vi "002 Panel Select.vi"(11 "Queue Ref In":T1={"UI"=refnum, "Message"=refnum, "Data"=refnum, "Caller"=refnum, "Name"="000 Common", "Data Path"=path "", "Class Path"=path "", "SubPanel"=refnum, "Project Name"="", "MNT"="", "Title"="", "Data Source"=refnum, "Queue List"={}, "VI"=refnum, "UE"=refnum}) -> ()   [LabVIEW 2020]
doc: "000001"
uses:
  Alin/QMH/000 Module Data Type.ctl
  Alin/QMH/Queue Message.ctl
  0007 Controls/Panel Select.ctl
  0007 Controls/Panel Element.ctl
  <vilib>/Utility/file.llb/Read Delimited Spreadsheet (string).vi
  <vilib>/Utility/file.llb/Write Delimited Spreadsheet (string).vi
panel:
  in  "Panel":T2
  in  "Edit":bool
  in  "Panel Left":bool
  in  "Help":bool
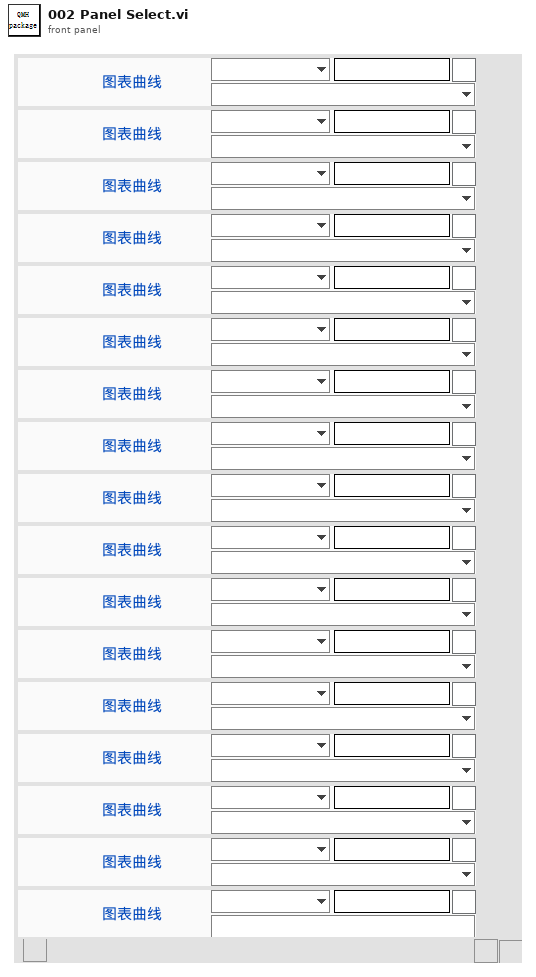
[diagram p1: front panel]
types:
  T1 = typedef "000 Module Data Type.ctl" = cluster{"UI":refnum<queue>, "Message":refnum<queue>, "Data":refnum<queue>, "Caller":refnum<queue>, "Name":string, "Data Path":path, "Class Path":path, "SubPanel":refnum<vi>, "Project Name":string, "MNT":string, "Title":string, "Data Source":refnum<queue>, "Queue List":map{string, refnum<queue>}, "VI":refnum<vi>, "UE":refnum<user-event>}
  T2 = typedef "Panel Select.ctl" = cluster{"Panel01":T3, "Panel02":T3, "Panel03":T3, "Panel01 2":T3, "Panel01 3":T3, "Panel01 4":T3, "Panel01 5":T3, "Panel01 6":T3, "Panel01 7":T3, "Panel01 8":T3, "Panel01 9":T3, "Panel01 10":T3, "Panel01 11":T3, "Panel01 12":T3, "Panel01 13":T3, "Panel01 14":T3, "Panel01 15":T3}
  T3 = typedef "Panel Element.ctl" = cluster{"BG":picture, "BTN":bool, "Panel":u16, "Name":string, "Use":bool, "BGSelect":u16}
  T4 = cluster{"Queue":T1, "Panel":T2, "Panels":string[], "BGs":string[], "Show?":bool, "PanelRef":refnum<vi>}
  T5 = cluster{"[0]":T3, "[1]":T3, "[2]":T3, "[3]":T3, "[4]":T3, "[5]":T3, "[6]":T3, "[7]":T3, "[8]":T3, "[9]":T3, "[10]":T3, "[11]":T3, "[12]":T3, "[13]":T3, "[14]":T3, "[15]":T3, "[16]":T3}
  T6 = typedef "imagedata.ctl" = cluster{"image type":i32, "image depth":i32, "image":u8[], "mask":u8[], "colors":u32[], "Rectangle":cluster{"left":i16, "top":i16, "right":i16, "bottom":i16}}
  T7 = typedef "eventvkey.ctl" = enum16{"ASCII", "Enter", "Return", "Shift", "Ctrl", "Alt", "Cmd", "Opt", "Caps", "NumLock", "Clear", "Break", "Up", "Down", "Left", "Right", "Insert", "Delete", "Home", "End", "PageUp", "PageDown", "Escape", "Help", "Pause", "ScrollLock", "F1", "F2", "F3", "F4", "F5", "F6", "F7", "F8", "F9", "F10", "F11", "F12", "F13", "F14", "F15", "F16", "F17", "F18", "F19", "F20", "F21", "F22", "F23", "F24", "Play", "VolumeUp", "VolumeDown", "Mute", "Two Byte Char"}
  T8 = cluster{"Shift":bool, "Ctrl":bool, "Alt":bool, "Cmd":bool, "Opt":bool}
  T9 = cluster{"Panel01":cluster{"BG":bool, "BTN":bool, "Panel":bool, "Name":bool, "Use":bool, "BGSelect":bool}, "Panel02":cluster{"BG":bool, "BTN":bool, "Panel":bool, "Name":bool, "Use":bool, "BGSelect":bool}, "Panel03":cluster{"BG":bool, "BTN":bool, "Panel":bool, "Name":bool, "Use":bool, "BGSelect":bool}, "Panel01 2":cluster{"BG":bool, "BTN":bool, "Panel":bool, "Name":bool, "Use":bool, "BGSelect":bool}, "Panel01 3":cluster{"BG":bool, "BTN":bool, "Panel":bool, "Name":bool, "Use":bool, "BGSelect":bool}, "Panel01 4":cluster{"BG":bool, "BTN":bool, "Panel":bool, "Name":bool, "Use":bool, "BGSelect":bool}, "Panel01 5":cluster{"BG":bool, "BTN":bool, "Panel":bool, "Name":bool, "Use":bool, "BGSelect":bool}, "Panel01 6":cluster{"BG":bool, "BTN":bool, "Panel":bool, "Name":bool, "Use":bool, "BGSelect":bool}, "Panel01 7":cluster{"BG":bool, "BTN":bool, "Panel":bool, "Name":bool, "Use":bool, "BGSelect":bool}, "Panel01 8":cluster{"BG":bool, "BTN":bool, "Panel":bool, "Name":bool, "Use":bool, "BGSelect":bool}, "Panel01 9":cluster{"BG":bool, "BTN":bool, "Panel":bool, "Name":bool, "Use":bool, "BGSelect":bool}, "Panel01 10":cluster{"BG":bool, "BTN":bool, "Panel":bool, "Name":bool, "Use":bool, "BGSelect":bool}, "Panel01 11":cluster{"BG":bool, "BTN":bool, "Panel":bool, "Name":bool, "Use":bool, "BGSelect":bool}, "Panel01 12":cluster{"BG":bool, "BTN":bool, "Panel":bool, "Name":bool, "Use":bool, "BGSelect":bool}, "Panel01 13":cluster{"BG":bool, "BTN":bool, "Panel":bool, "Name":bool, "Use":bool, "BGSelect":bool}, "Panel01 14":cluster{"BG":bool, "BTN":bool, "Panel":bool, "Name":bool, "Use":bool, "BGSelect":bool}, "Panel01 15":cluster{"BG":bool, "BTN":bool, "Panel":bool, "Name":bool, "Use":bool, "BGSelect":bool}}
  T10 = cluster{"BG":bool, "BTN":bool, "Panel":bool, "Name":bool, "Use":bool, "BGSelect":bool}[]
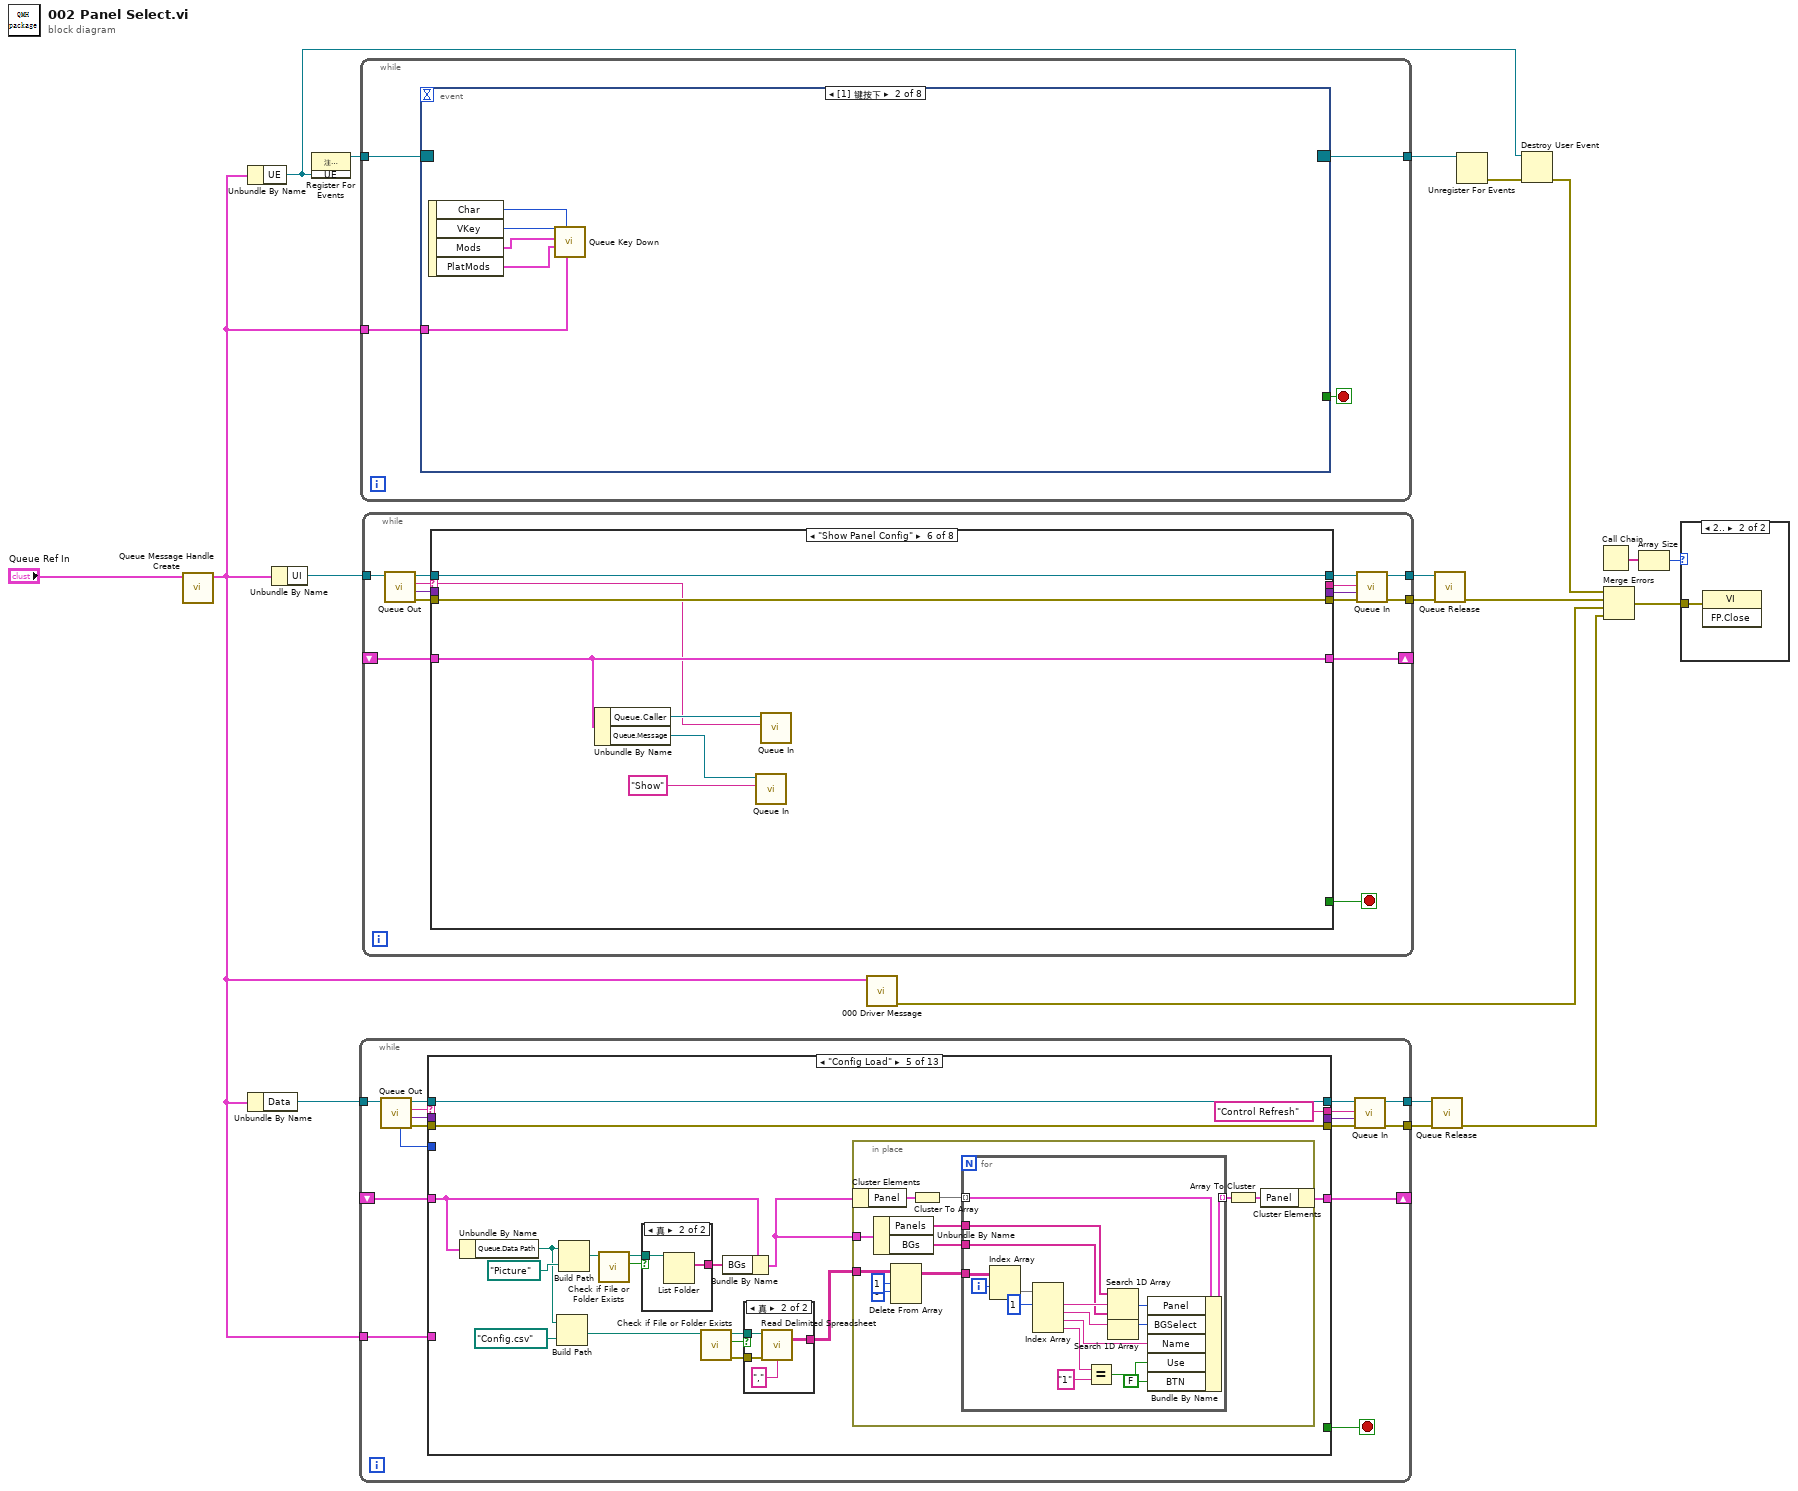
[diagram p0: block diagram]
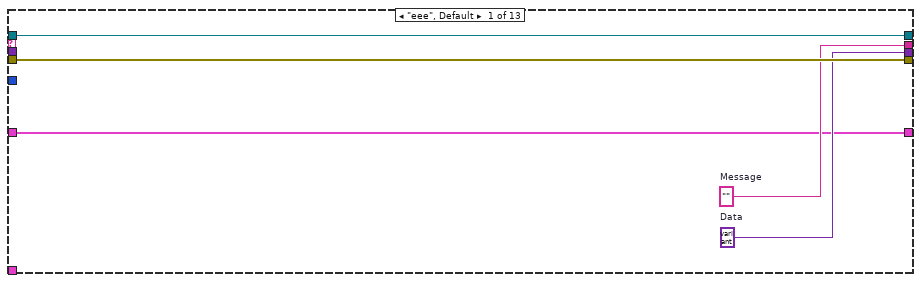
[diagram p2: hidden frame]
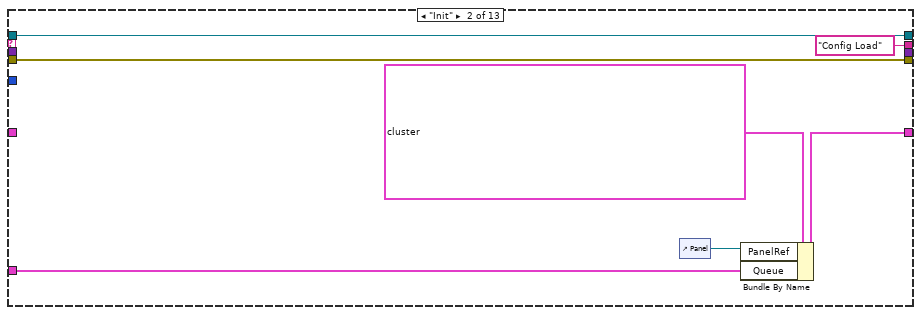
[diagram p3: hidden frame]
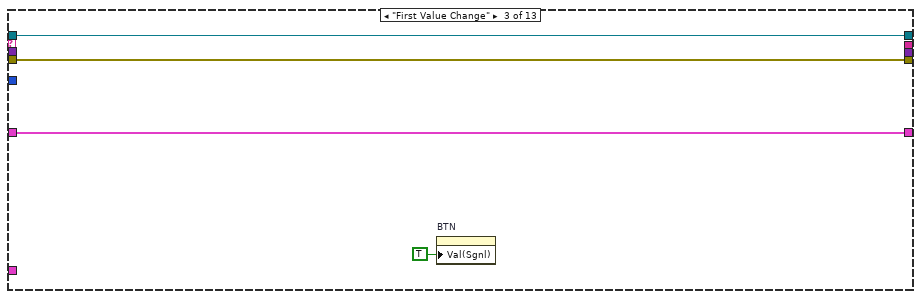
[diagram p4: hidden frame]
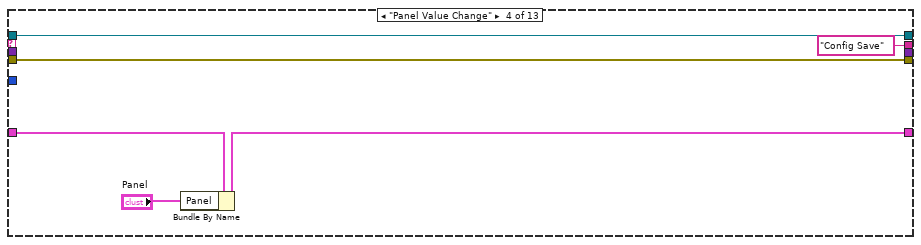
[diagram p5: hidden frame]
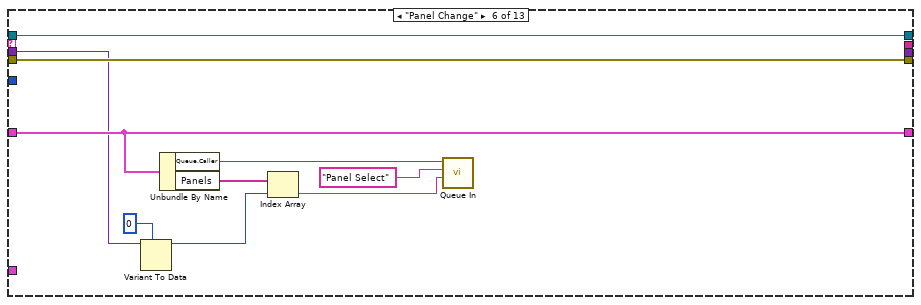
[diagram p8: hidden frame]
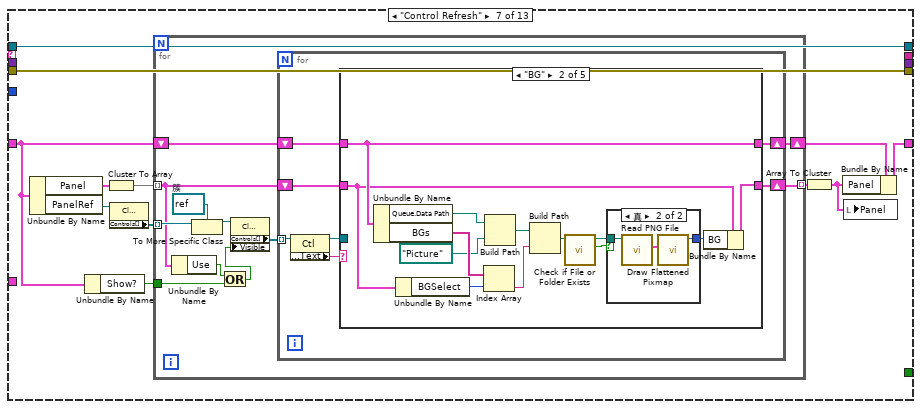
[diagram p9: hidden frame]
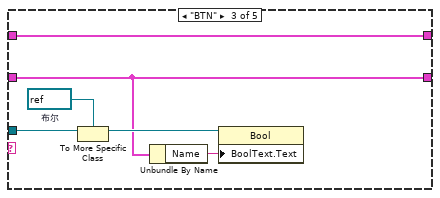
[diagram p12: hidden frame]
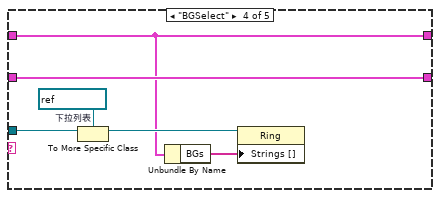
[diagram p13: hidden frame]
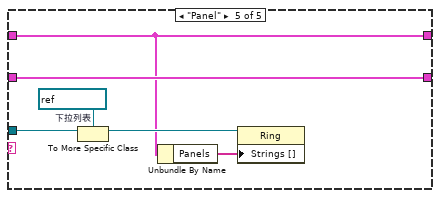
[diagram p14: hidden frame]
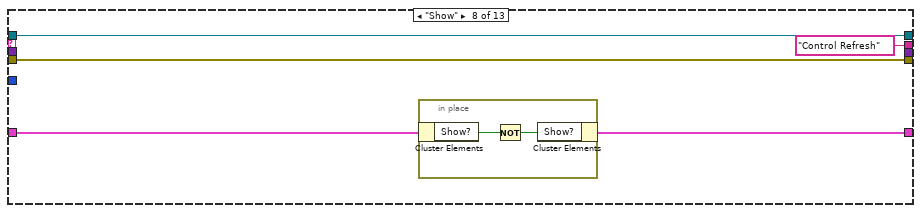
[diagram p15: hidden frame]
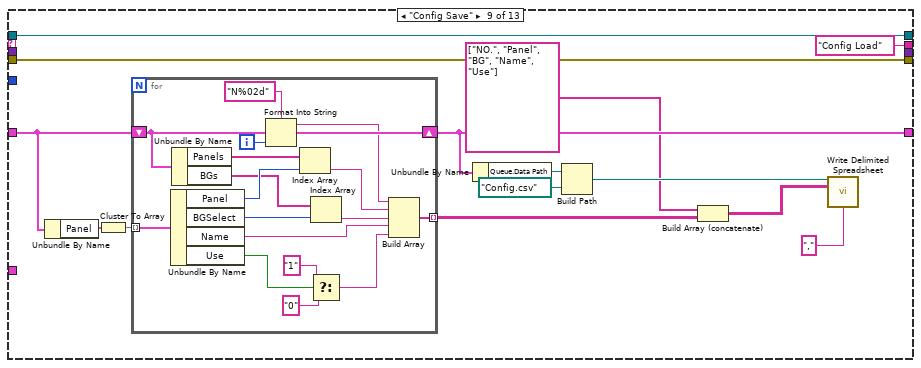
[diagram p16: hidden frame]
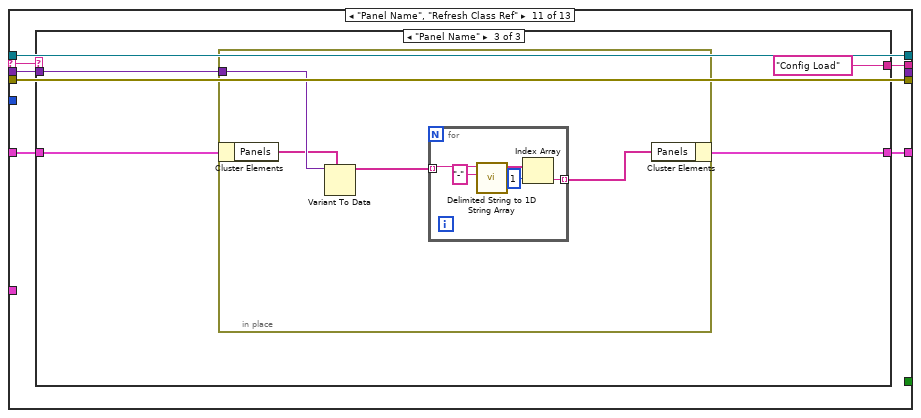
[diagram p18: hidden frame]
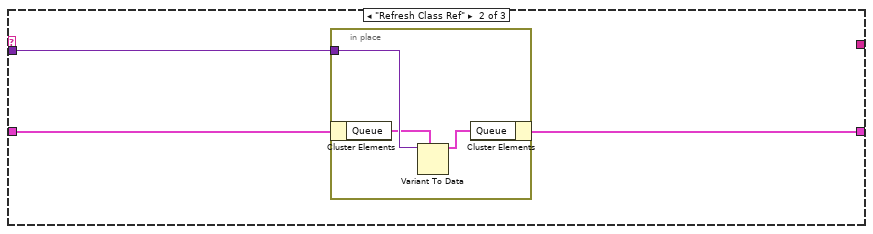
[diagram p20: hidden frame]
diagram:
  n1 = call "Queue Message Handle Create.vi"("Queue Ref In"="Queue Ref In") -> ("Queue Ref Out"=w1:T1)  [unwired: 9 in, 1 out]
  n2 = Unbundle By Name(w1) -> ("UE"=w3:refnum<user-event>)
  n3 = Unbundle By Name(w1) -> ("Data"=w6:refnum<queue>)
  n4 = Unbundle By Name(w1) -> ("UI"=w14:refnum<queue>)
  n5 = register-events(w3) -> (reference out=w19:refnum<event-registration>)  [unwired: 2 in, 1 out]
  n6 = while {
    tunnel: w6 -> [w31]
    tunnel: [w28] -> w8
    tunnel: [w27] -> w7
    shift-right: [w23] -> _
    shift-left: _ -> [w22]
    tunnel: w1 -> [w20]
    stop <- w35 stop-if-true
    n7 = call "Queue Out.vi"("Queue In"=w31) -> ("error out"=w34:errorcluster, "Data"=w32:variant, "Message"=w33:string, "Queue Out"=w30:refnum<queue>, "Queue NUmber"=w21:i32)  [unwired: 6 in]
    n8 = case shown="\"Config Load\"" w33 {
      selector: w33 -> [_ _ _ _ _ _ _ _ _ _ w228 _ _]
      tunnel: w30 -> [w40 w47 w51 w57 w75 w119 w131 w190 w206 w226 w233 w258 w262]
      tunnel: w34 -> [w39 w46 w50 w56 w74 w118 w130 w189 w205 w225 w232 w256 w263]
      tunnel: [w40 w47 w51 w57 w75 w119 w131 w190 w206 w226 w233 w257 w262] -> w29
      tunnel: [w39 w46 w50 w56 w74 w118 w130 w189 w205 w225 w232 w255 w263] -> w26
      tunnel: [w38 "Config Load" ("Message") _ "Config Save" ("Message") "Control Refresh" ("Message") _ _ "Control Refresh" ("Message") "Config Load" ("Message") _ w227 "Quit" _] -> w25
      tunnel: [_ _ _ _ _ _ _ _ _ _ _ _ TRUE] -> w35
      tunnel: [w37 _ _ _ _ _ _ _ _ _ _ _ _] -> w24
      tunnel: w32 -> [_ _ _ _ _ w116 _ _ _ _ w229 _ _]
      tunnel: [w36 w44 w49 w54 w66 w117 w125 w187 w198 w224 w230 w254 w260] -> w23
      tunnel: w22 -> [w36 _ w49 w55 w73 w117 w121 w188 w201 w224 w231 w254 w260]
      tunnel: w21 -> [_ _ _ _ _ _ _ _ _ _ _ _ _]
      tunnel: w20 -> [_ w42 _ _ _ _ _ _ _ _ _ _ _]
      frame "eee", Default {
        w37 = variant  # Data
        w38 = ""  # Message
      }
      frame "Init" {
        n9 = control-ref of="Panel"() -> (w41:refnum<vi>)
        n10 = Bundle By Name(cluster=T4 {"Queue"={"UI"=refnum, "Message"=refnum, "Data"=refnum, "Caller"=refnum, "Name"="000 Common", "Data Path"=path "", "Class Path"=path "", "SubPanel"=refnum, "Project Name"="", "MNT"="", "Title"="", "Data Source"=refnum, "Queue List"={}, "VI"=refnum, "UE"=refnum}, "Panel"={"Panel01"={"BG"=bytes[0], "BTN"=TRUE, "Panel"=0, "Name"="", "Use"=FALSE, "BGSelect"=0}, "Panel02"={"BG"=bytes[0], "BTN"=TRUE, "Panel"=0, "Name"="", "Use"=FALSE, "BGSelect"=0}, "Panel03"={"BG"=bytes[0], "BTN"=FALSE, "Panel"=0, "Name"="", "Use"=FALSE, "BGSelect"=0}, "Panel01 2"={"BG"=bytes[0], "BTN"=FALSE, "Panel"=0, "Name"="", "Use"=FALSE, "BGSelect"=0}, "Panel01 3"={"BG"=bytes[0], "BTN"=FALSE, "Panel"=0, "Name"="", "Use"=FALSE, "BGSelect"=0}, "Panel01 4"={"BG"=bytes[0], "BTN"=FALSE, "Panel"=0, "Name"="", "Use"=FALSE, "BGSelect"=0}, "Panel01 5"={"BG"=bytes[0], "BTN"=FALSE, "Panel"=0, "Name"="", "Use"=FALSE, "BGSelect"=0}, "Panel01 6"={"BG"=bytes[0], "BTN"=FALSE, "Panel"=0, "Name"="", "Use"=FALSE, "BGSelect"=0}, "Panel01 7"={"BG"=bytes[0], "BTN"=FALSE, "Panel"=0, "Name"="", "Use"=FALSE, "BGSelect"=0}, "Panel01 8"={"BG"=bytes[0], "BTN"=FALSE, "Panel"=0, "Name"="", "Use"=FALSE, "BGSelect"=0}, "Panel01 9"={"BG"=bytes[0], "BTN"=FALSE, "Panel"=0, "Name"="", "Use"=FALSE, "BGSelect"=0}, "Panel01 10"={"BG"=bytes[0], "BTN"=FALSE, "Panel"=0, "Name"="", "Use"=FALSE, "BGSelect"=0}, "Panel01 11"={"BG"=bytes[0], "BTN"=FALSE, "Panel"=0, "Name"="", "Use"=FALSE, "BGSelect"=0}, "Panel01 12"={"BG"=bytes[0], "BTN"=FALSE, "Panel"=0, "Name"="", "Use"=FALSE, "BGSelect"=0}, "Panel01 13"={"BG"=bytes[0], "BTN"=FALSE, "Panel"=0, "Name"="", "Use"=FALSE, "BGSelect"=0}, "Panel01 14"={"BG"=bytes[0], "BTN"=FALSE, "Panel"=0, "Name"="", "Use"=FALSE, "BGSelect"=0}, "Panel01 15"={"BG"=bytes[0], "BTN"=FALSE, "Panel"=0, "Name"="", "Use"=FALSE, "BGSelect"=0}}, "Panels"=[], "BGs"=[], "Show?"=FALSE, "PanelRef"=refnum}, "PanelRef"=w41, "Queue"=w42) -> (w44:T4)
      }
      frame "First Value Change" {
        n11 = property on="BTN" class="Bool (严格)"("Val(Sgnl)"=TRUE ("值(信号)")) -> ()  [unwired: 2 in, 2 out]
      }
      frame "Panel Value Change" {
        n12 = Bundle By Name(cluster=w55, "Panel"="Panel") -> (w54:T4)
      }
      frame "Config Load" {
        n13 = Unbundle By Name(w73) -> ("Queue.Data Path"=w64:path)
        n14 = Build Path(base path=w64, name or relative path=path "Config.csv" ("名称或相对路径")) -> (appended path=w58:path)
        n15 = Build Path(base path=w64, name or relative path=path "Picture" ("名称或相对路径")) -> (appended path=w70:path)
        n16 = call <vilib>:"Check if File or Folder Exists.vi"("path"=w70) -> ("file or folder exists?"=w68:bool, "dup path"=w69:path)  [unwired: 8 in, 1 out]
        n17 = case shown="真" w68 {
          tunnel: [_ w109] -> w71
          tunnel: w69 -> [_ w108]
          frame False {
          }
          frame True {
            n18 = List Folder(path=w108) -> (filenames=w109:string[])  [unwired: 3 in, 3 out]
          }
        }
        n19 = call <vilib>:"Check if File or Folder Exists.vi"("path"=w58) -> ("error out"=w60:errorcluster, "file or folder exists?"=w62:bool, "dup path"=w61:path)  [unwired: 8 in]
        n20 = Bundle By Name(cluster=w73, "BGs"=w71) -> (w65:T4)
        n21 = case shown="真" w62 {
          tunnel: w61 -> [_ w78]
          tunnel: w60 -> [_ w77]
          tunnel: [_ w76] -> w59
          frame False {
          }
          frame True {
            n22 = call-poly <vilib>:"Read Delimited Spreadsheet.vi"("file path (dialog if empty)"=w78, "error in (no error)"=w77, "delimiter (\\t)"="," ("delimiter (\\t)")) -> ("all rows"=w76:string[][])  [unwired: 7 in, 5 out]
          }
        }
        n23 = in-place {
          in-place-border: w59 -> [w90]
          in-place-border: w65 -> [w82]
          n24 = in-place-cluster #1(w65) -> ("Panel"=w87:T2)
          n25 = Unbundle By Name(w82) -> ("Panels"=w81:string[], "BGs"=w80:string[])
          n26 = Delete From Array(array=w90, length=1 ("长度"), index (row)=0 ("索引 (行)")) -> (array with subset deleted=w83:string[][])  [unwired: 1 in, 1 out]
          n27 = Cluster To Array(cluster=w87) -> (array=w86:T3[])
          n28 = for {
            tunnel: w86 -> [w107] mode=indexing
            tunnel: [w100] -> w85 mode=indexing
            tunnel: w83 -> [w106]
            tunnel: w81 -> [w102]
            tunnel: w80 -> [w98]
            i -> [w105]
            n29 = Index Array(array=w106, index (row)=w105) -> (element=w104:string[])  [unwired: 1 in]
            n30 = Index Array(array=w104, index #1=1 ("索引")) -> (element #1=w101:string, element #2=w97:string, element #3=w95:string, element #4=w94:string)  [unwired: 3 in]
            n31 = Equal?(x=w94, y="1") -> (x = y?=w92:bool)
            n32 = Search 1D Array(1D array=w102, element=w101) -> (index of element=w99:i32)  [unwired: 1 in]
            n33 = Search 1D Array(1D array=w98, element=w97) -> (index of element=w96:i32)  [unwired: 1 in]
            n34 = Bundle By Name(cluster=w107, "Panel"=w99, "BGSelect"=w96, "Name"=w95, "Use"=w92, "BTN"=FALSE) -> (w100:T3)
          }
          n35 = Array To Cluster(array=w85) -> (cluster=w84:T5)
          n36 = in-place-cluster #1("Panel"=w84) -> (w66:T4)
        }
      }
      frame "Panel Change" {
        n37 = Variant To Data(type=u16 0 ("Panel"), Variant=w116) -> (data=w113:u16)  [unwired: 1 in, 1 out]
        n38 = Unbundle By Name(w117) -> ("Queue.Caller"=w112:refnum<queue>, "Panels"=w114:string[])
        n39 = Index Array(array=w114, index=w113) -> (element=w110:string)
        n40 = call "Queue In.vi"("Data"=w110, "Message"="Panel Select", "Queue In"=w112) -> ()  [unwired: 7 in, 2 out]
      }
      frame "Control Refresh" {
        n41 = Unbundle By Name(w121) -> ("Panel"=w127:T2, "PanelRef"=w129:refnum<vi>)
        n42 = Unbundle By Name(w121) -> ("Show?"=w120:bool)
        n43 = Cluster To Array(cluster=w127) -> (array=w126:T3[])
        n44 = property class="Clust"(reference=w129) -> ("Controls[]"=w128:refnum<vi>[])  [unwired: 1 in, 2 out]
        n45 = for {
          tunnel: w128 -> [w139] mode=indexing
          tunnel: w126 -> [w135] mode=indexing
          tunnel: [w142] -> w124 mode=indexing
          shift-right: [w140] -> w123
          shift-left: w121 -> [w141]
          tunnel: w120 -> [w133]
          w138 = refnum<vi> refnum  # 簇
          n46 = Unbundle By Name(w135) -> ("Use"=w134:bool)
          n47 = To More Specific Class(target class=w138, reference=w139) -> (specific class reference=w137:refnum<vi>)  [unwired: 1 in, 1 out]
          n48 = Or(x=w134, y=w133) -> (x .or. y?=w132:bool)
          n49 = property class="Clust"(reference=w137, "Visible"=w132) -> ("Controls[]"=w136:refnum<vi>[])  [unwired: 1 in, 2 out]
          n50 = for {
            shift-right: [w148] -> w142
            shift-left: w135 -> [w149]
            shift-right: [w146] -> w140
            shift-left: w141 -> [w147]
            tunnel: w136 -> [w145] mode=indexing
            n51 = property class="Ctl"(reference=w145) -> (reference out=w143:refnum<vi>, "Label.Text"=w144:string)  [unwired: 1 in, 1 out]
            n52 = case shown="\"BG\"" w144 {
              tunnel: w149 -> [w151 w163 w169 w178 w184]
              tunnel: [w151 w162 w169 w178 w184] -> w148
              tunnel: w147 -> [w150 w164 w173 w175 w181]
              tunnel: [w150 w164 w173 w175 w181] -> w146
              tunnel: w143 -> [_ _ w172 w179 w185]
              frame Default {
              }
              frame "BG" {
                n53 = Unbundle By Name(w164) -> ("Queue.Data Path"=w159:path, "BGs"=w161:string[])
                n54 = Unbundle By Name(w163) -> ("BGSelect"=w160:u16)
                n55 = Index Array(array=w161, index=w160) -> (element=w155:string)
                n56 = Build Path(base path=w159, name or relative path=path "Picture" ("名称或相对路径")) -> (appended path=w156:path)
                n57 = Build Path(base path=w156, name or relative path=w155) -> (appended path=w154:path)
                n58 = call <vilib>:"Check if File or Folder Exists.vi"("path"=w154) -> ("file or folder exists?"=w152:bool, "dup path"=w153:path)  [unwired: 8 in, 1 out]
                n59 = case shown="真" w152 {
                  tunnel: [_ w166] -> w158
                  tunnel: w153 -> [_ w165]
                  frame False {
                  }
                  frame True {
                    n60 = call <vilib>:"Read PNG File.vi"("path to PNG file"=w165) -> ("image data"=w167:T6)  [unwired: 8 in, 2 out]
                    n61 = call <vilib>:"Draw Flattened Pixmap.vi"("image data"=w167) -> ("new picture"=w166:picture)  [unwired: 8 in]
                  }
                }
                n62 = Bundle By Name(cluster=w163, "BG"=w158) -> (w162:T3)
              }
              frame "BTN" {
                w171 = refnum<vi> refnum  # 布尔
                n63 = To More Specific Class(target class=w171, reference=w172) -> (specific class reference=w170:refnum<vi>)  [unwired: 1 in, 1 out]
                n64 = Unbundle By Name(w169) -> ("Name"=w168:string)
                n65 = property class="Bool"(reference=w170, "BoolText.Text"=w168) -> ()  [unwired: 1 in, 2 out]
              }
              frame "BGSelect" {
                w176 = refnum<vi> refnum  # 下拉列表
                n66 = To More Specific Class(target class=w176, reference=w179) -> (specific class reference=w177:refnum<vi>)  [unwired: 1 in, 1 out]
                n67 = Unbundle By Name(w175) -> ("BGs"=w174:string[])
                n68 = property class="Ring"(reference=w177, "Strings []"=w174) -> ()  [unwired: 1 in, 2 out]
              }
              frame "Panel" {
                w182 = refnum<vi> refnum  # 下拉列表
                n69 = To More Specific Class(target class=w182, reference=w185) -> (specific class reference=w183:refnum<vi>)  [unwired: 1 in, 1 out]
                n70 = Unbundle By Name(w181) -> ("Panels"=w180:string[])
                n71 = property class="Ring"(reference=w183, "Strings []"=w180) -> ()  [unwired: 1 in, 2 out]
              }
            }
          }
        }
        n72 = Array To Cluster(array=w124) -> (cluster=w122:T5)
        n73 = Bundle By Name(cluster=w123, "Panel"=w122) -> (w125:T4)
        n74 = local write "Panel"(w122) -> ()
      }
      frame "Show" {
        n75 = in-place {
          n76 = in-place-cluster #2(w188) -> ("Show?"=w192:bool)
          n77 = Not(x=w192) -> (.not. x?=w191:bool)
          n78 = in-place-cluster #2("Show?"=w191) -> (w187:T4)
        }
      }
      frame "Config Save" {
        n79 = Unbundle By Name(w201) -> ("Panel"=w204:T2)
        n80 = Cluster To Array(cluster=w204) -> (array=w203:T3[])
        n81 = for {
          tunnel: w203 -> [w223] mode=indexing
          shift-right: [w217] -> w198
          shift-left: w201 -> [w217]
          tunnel: [w207] -> w194 mode=indexing
          i -> [w215]
          n82 = Unbundle By Name(w223) -> ("Panel"=w219:u16, "BGSelect"=w212:u16, "Name"=w210:string, "Use"=w209:bool)
          n83 = Unbundle By Name(w217) -> ("Panels"=w220:string[], "BGs"=w213:string[])
          n84 = Format Into String(format string="N%02d" ("格式字符串"), w215) -> (resulting string=w214:string)  [unwired: 2 in, 1 out]
          n85 = Index Array(array=w220, index=w219) -> (element=w218:string)
          n86 = Index Array(array=w213, index=w212) -> (element=w211:string)
          n87 = Select(t="1", s=w209, f="0") -> (s? t:f=w208:string)
          n88 = Build Array(w214, w218, w211, w210, w208) -> (w207:string[])
        }
        n89 = Unbundle By Name(w198) -> ("Queue.Data Path"=w199:path)
        n90 = Build Path(base path=w199, name or relative path=path "Config.csv" ("名称或相对路径")) -> (appended path=w197:path)
        n91 = Build Array (concatenate)(string[] ["NO.", "Panel", "BG", "Name", "Use"], w194) -> (w193:string[][])
        n92 = call-poly <vilib>:"Write Delimited Spreadsheet.vi"("file path (dialog if empty)"=w197, "2D data"=w193, "delimiter (\\t)"="," ("delimiter (\\t)")) -> ()  [unwired: 11 in, 2 out]
      }
      frame "====System====" {
      }
      frame "Panel Name", "Refresh Class Ref" {
        n93 = case shown="\"Panel Name\"" w228 {
          tunnel: w231 -> [w234 w237 w244]
          tunnel: [w234 w236 w243] -> w230
          tunnel: w229 -> [_ w235 w242]
          tunnel: [_ _ "Config Load"] -> w227
          frame "eee", Default {
          }
          frame "Refresh Class Ref" {
            n94 = in-place {
              in-place-border: w235 -> [w240]
              n95 = in-place-cluster #3(w237) -> ("Queue"=w239:T1)
              n96 = Variant To Data(type=w239, Variant=w240) -> (data=w238:T1)  [unwired: 1 in, 1 out]
              n97 = in-place-cluster #3("Queue"=w238) -> (w236:T4)
            }
          }
          frame "Panel Name" {
            n98 = in-place {
              in-place-border: w242 -> [w248]
              n99 = in-place-cluster #4(w244) -> ("Panels"=w247:string[])
              n100 = Variant To Data(type=w247, Variant=w248) -> (data=w246:string[])  [unwired: 1 in, 1 out]
              n101 = for {
                tunnel: w246 -> [w253] mode=indexing
                tunnel: [w249] -> w245 mode=indexing
                n102 = call <vilib>:"Delimited String to 1D String Array.vi"("delimiter"="-", "delimited string"=w253) -> ("string array"=w251:string[])  [unwired: 9 in]
                n103 = Index Array(array=w251, index=1 ("索引")) -> (element=w249:string)
              }
              n104 = in-place-cluster #4("Panels"=w245) -> (w243:T4)
            }
          }
        }
      }
      frame "Exit" {
        n105 = call "Queue Clear.vi"("error in (no error)"=w256, "Queue In"=w258) -> ("error out"=w255:errorcluster, "Queue Out"=w257:refnum<queue>)  [unwired: 8 in]
      }
      frame "Quit" {
      }
    }
    n106 = call "Queue In.vi"("error in (no error)"=w26, "Data"=w24, "Message"=w25, "Queue In"=w29) -> ("error out"=w27:errorcluster, "Queue Out"=w28:refnum<queue>)  [unwired: 6 in]
  }
  n107 = while {
    tunnel: w19 -> [w267]
    tunnel: [w265] -> w18
    tunnel: w1 -> [w264]
    stop <- w266 stop-if-true
    n108 = event shown="[1] 键按下" {
      selector: w267 -> [_ _ _ _ _ _ _ _]
      dyn-events: [_ _ _ _ _ _ _ _] -> w265
      timeout: _ -> [_ _ _ _ _ _ _ _]
      tunnel: [_ _ w273 _ _ _ _ _] -> w266
      tunnel: w264 -> [_ w270 _ w278 w296 w319 w324 w328]
      event Timeout {
        n109 = event-data() -> ()  [unwired: 1 in, 1 out]
      }
      event Key Down {
        n110 = event-data() -> ("Char"=w272:i16, "VKey"=w271:T7, "Mods"=w269:cluster{"Num Pad":bool, "Menu Key":bool}, "PlatMods"=w268:T8)  [unwired: 1 in]
        n111 = call "Queue Key Down.vi"("Queue Ref Out"=w270, "C"=w272, "Platform Key"=w268, "Group Key"=w269, "V Key"=w271) -> ()  [unwired: 6 in, 1 out]
      }
      event User Event {
        n112 = event-data() -> ("Message"=w275:string)  [unwired: 1 in]
        n113 = Equal?(x=w275, y="Exit") -> (x = y?=w273:bool)
      }
      event Panel Close? {
        n114 = event-data() -> ()  [unwired: 1 in, 1 out]
        n115 = Call Chain() -> (call chain=w280:string[])
        n116 = Array Size(array=w280) -> (size(s)=w279:i32)
        n117 = case shown="2, 默认" w279 {
          tunnel: w278 -> [w284 w287]
          tunnel: [w283 w286] -> w277
          tunnel: ["Panel Hidden" ("Message") "Exit Prepare" ("Message")] -> w276
          frame 2, Default {
            n118 = Unbundle By Name(w284) -> ("Message"=w283:refnum<queue>)
          }
          frame 1 {
            n119 = Unbundle By Name(w287) -> ("Message"=w286:refnum<queue>)
          }
        }
        n120 = call "Queue In.vi"("Message"=w276, "Queue In"=w277) -> ()  [unwired: 8 in, 2 out]
        n121 = event-data("Discard?"=TRUE ("放弃？")) -> ()  [unwired: 1 in, 1 out]
      }
      event Value Change {
        n122 = event-data() -> ("NewVal"=w294:T2, "OldVal"=w295:T2)  [unwired: 1 in]
        n123 = flat-sequence {
          tunnel: w296 -> [w302]
          tunnel: w295 -> [w309]
          tunnel: w294 -> [w306]
          tunnel: [w302] -> w290
          tunnel: [w301] -> w293
          tunnel: [w300] -> w292
          frame #0 {
            n124 = Not Equal?(x=w306, y=w309) -> (x != y?=w308:T9)
            n125 = Cluster To Array(cluster=w308) -> (array=w307:T10)
            n126 = Cluster To Array(cluster=w306) -> (array=w305:T3[])
            n127 = for {
              tunnel: w307 -> [w316] mode=indexing
              tunnel: w305 -> [w313] mode=indexing
              tunnel: [w312] -> w304 mode=indexing
              tunnel: [w310] -> w301 if=w310
              tunnel: [w311] -> w300 if=w310
              n128 = Unbundle By Name(w313) -> ("Panel"=w311:u16, "BTN"=w315:bool)
              n129 = Unbundle By Name(w316) -> ("BTN"=w314:bool)
              n130 = And(x=w315, y=w314) -> (x .and. y?=w310:bool)
              n131 = Bundle By Name(cluster=w313, "BTN"=w310) -> (w312:T3)
            }
            n132 = Array To Cluster(array=w304) -> (cluster=w303:T5)
            n133 = local write "Panel"(w303) -> ()
          }
        }
        n134 = case shown="真" w293 {
          tunnel: w292 -> [w297 _]
          tunnel: ["Panel Change" ("Message") "Panel Value Change" ("Message")] -> w289
          tunnel: [w297 _] -> w288
          frame True {
          }
          frame False {
          }
        }
        n135 = Unbundle By Name(w290) -> ("Data"=w291:refnum<queue>)
        n136 = call "Queue In.vi"("Data"=w288, "Message"=w289, "Queue In"=w291) -> ()  [unwired: 7 in, 2 out]
      }
      event "Edit": Value Change {
        n137 = event-data() -> ()  [unwired: 1 in, 1 out]
        n138 = Unbundle By Name(w319) -> ("UI"=w318:refnum<queue>)
        n139 = call "Queue In.vi"("Message"="Show Panel Config", "Queue In"=w318) -> ()  [unwired: 8 in, 2 out]
      }
      event "Panel Left": Value Change {
        n140 = event-data() -> ("CtlRef"=w323:refnum<vi>)  [unwired: 1 in]
        n141 = Unbundle By Name(w324) -> ("Caller"=w322:refnum<queue>)
        n142 = property class="Bool (严格)"(reference=w323) -> ("Label.Text"=w321:string)  [unwired: 1 in, 2 out]
        n143 = call "Queue In.vi"("Data"="Panel Left", "Message"=w321, "Queue In"=w322) -> ()  [unwired: 7 in, 2 out]
      }
      event "Help": Value Change {
        n144 = event-data() -> ("CtlRef"=w326:refnum<vi>)  [unwired: 1 in]
        n145 = Unbundle By Name(w328) -> ("UI"=w327:refnum<queue>)
        n146 = property class="Bool"(reference=w326) -> ("Label.Text"=w325:string)  [unwired: 1 in, 2 out]
        n147 = call "Queue In.vi"("Message"=w325, "Queue In"=w327) -> ()  [unwired: 8 in, 2 out]
      }
    }
  }
  n148 = while {
    tunnel: w14 -> [w338]
    tunnel: [w335] -> w16
    tunnel: [w334] -> w15
    shift-right: [w330] -> _
    shift-left: _ -> [w329]
    stop <- w342 stop-if-true
    n149 = call "Queue Out.vi"("Queue In"=w338) -> ("error out"=w341:errorcluster, "Data"=w339:variant, "Message"=w340:string, "Queue Out"=w337:refnum<queue>)  [unwired: 6 in, 1 out]
    n150 = case shown="\"Show Panel Config\"" w340 {
      selector: w340 -> [_ _ _ _ w357 w377 w384 _]
      tunnel: w337 -> [w347 w350 w353 w356 w362 w381 w391 w397]
      tunnel: w341 -> [w346 w349 w352 w355 w361 w380 w389 w398]
      tunnel: [w347 w350 w353 w356 w362 w381 w390 w397] -> w336
      tunnel: [w346 w349 w352 w355 w361 w380 w388 w398] -> w333
      tunnel: [w345 _ _ _ _ _ "Quit" _] -> w332
      tunnel: [_ _ _ _ _ _ _ TRUE] -> w342
      tunnel: [w344 _ _ _ _ _ _ _] -> w331
      tunnel: w339 -> [_ _ _ _ w358 _ _ _]
      tunnel: [w343 cluster{"Queue":T1} {"Queue"={"UI"=refnum, "Message"=refnum, "Data"=refnum, "Caller"=refnum, "Name"="000 Common", "Data Path"=path "", "Class Path"=path "", "SubPanel"=refnum, "Project Name"="", "MNT"="", "Title"="", "Data Source"=refnum, "Queue List"={}, "VI"=refnum, "UE"=refnum}} w351 w354 w359 w379 w383 w395] -> w330
      tunnel: w329 -> [w343 _ w351 w354 w360 w379 w383 w395]
      frame "eee", Default {
        w344 = variant  # Data
        w345 = ""  # Message
      }
      frame "Init" {
      }
      frame "Help" {
      }
      frame "====System====" {
      }
      frame "Refresh Class Ref" {
        n151 = case shown="\"Refresh Class Ref\"" w357 {
          tunnel: w360 -> [w363 w368]
          tunnel: [w363 w366] -> w359
          tunnel: w358 -> [_ w367]
          frame "eee", Default {
          }
          frame "Refresh Class Ref" {
            n152 = in-place {
              in-place-border: w367 -> [w374]
              n153 = in-place-cluster #5(w368) -> ("Queue"=w373:T1)
              n154 = Variant To Data(type=w373, Variant=w374) -> (data=w372:T1)  [unwired: 1 in, 1 out]
              n155 = in-place-cluster #5("Queue"=w372) -> (w366:cluster{"Queue":T1})
            }
            n156 = Call Chain() -> (call chain=w365:string[])
            n157 = Array Size(array=w365) -> (size(s)=w364:i32)
            n158 = case shown="2.." w364 {
              tunnel: w366 -> [_ w371]
              frame 0, Default {
              }
              frame 2.. {
                n159 = Unbundle By Name(w371) -> ("Queue.Message"=w370:refnum<queue>)
                n160 = call "Queue In.vi"("Message"="Panel Insert", "Queue In"=w370) -> ()  [unwired: 8 in, 2 out]
              }
            }
          }
        }
      }
      frame "Show Panel Config" {
        n161 = Unbundle By Name(w379) -> ("Queue.Caller"=w378:refnum<queue>, "Queue.Message"=w376:refnum<queue>)
        n162 = call "Queue In.vi"("Message"="Show", "Queue In"=w376) -> ()  [unwired: 8 in, 2 out]
        n163 = call "Queue In.vi"("Message"=w377, "Queue In"=w378) -> ()  [unwired: 8 in, 2 out]
      }
      frame "Exit" {
        n164 = Unbundle By Name(w383) -> ("Queue.Message"=w387:refnum<queue>, "Queue.Data"=w386:refnum<queue>, "Queue.UE"=w382:refnum<user-event>)
        n165 = Build Array(w387, w386) -> (w385:refnum<queue>[])
        n166 = Generate User Event(user event=w382, event data cluster=w384) -> ()  [unwired: 2 in, 2 out]
        n167 = for {
          tunnel: w385 -> [w394] mode=indexing
          tunnel: w384 -> [w393]
          n168 = call "Queue In.vi"("Message"=w393, "Queue In"=w394) -> ()  [unwired: 8 in, 2 out]
        }
        n169 = call "Queue Clear.vi"("error in (no error)"=w389, "Queue In"=w391) -> ("error out"=w388:errorcluster, "Queue Out"=w390:refnum<queue>)  [unwired: 8 in]
      }
      frame "Quit" {
      }
    }
    n170 = call "Queue In.vi"("error in (no error)"=w333, "Data"=w331, "Message"=w332, "Queue In"=w336) -> ("error out"=w334:errorcluster, "Queue Out"=w335:refnum<queue>)  [unwired: 6 in]
  }
  n171 = call "000 Driver Message.vi"("Queue In"=w1) -> ("error out"=w4:errorcluster)  [unwired: 8 in, 2 out]
  n172 = call "Queue Release.vi"("error in (no error)"=w7, "Queue In"=w8) -> ("error out"=w5:errorcluster)  [unwired: 9 in]
  n173 = call "Queue Release.vi"("error in (no error)"=w15, "Queue In"=w16) -> ("error out"=w12:errorcluster)  [unwired: 9 in]
  n174 = Unregister For Events(event registration refnum=w18) -> (error out=w17:errorcluster)  [unwired: 1 in]
  n175 = Destroy User Event(user event=w3, error in=w17) -> (error out=w13:errorcluster)
  n176 = Call Chain() -> (call chain=w10:string[])
  n177 = Merge Errors(w13, w12, w4, w5) -> (w11:errorcluster)
  n178 = Array Size(array=w10) -> (size(s)=w9:i32)
  n179 = case shown="2.." w9 {
    tunnel: w11 -> [_ w399]
    frame 0, Default {
    }
    frame 2.. {
      n180 = invoke class="VI" method="FP.Close"(error in=w399) -> ()  [unwired: 2 in, 3 out]
    }
  }
